vi "get_modelock_status.vi"(8 "error in (no error)":errorcluster, 11 "VISA resource name":refnum<visa-resource-name>) -> (0 "error out":errorcluster, 1 "color":u32, 2 "modelock (0,1,2=off,ML,CW)":i32, 3 "VISA resource name out":refnum<visa-resource-name>)   [LabVIEW 2013]
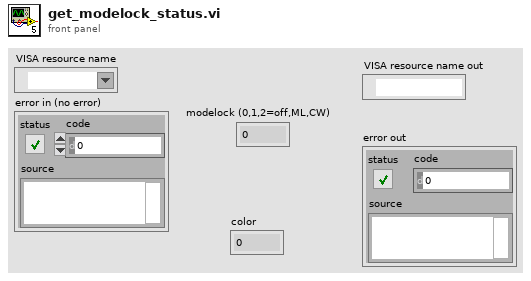
[diagram p1: front panel]
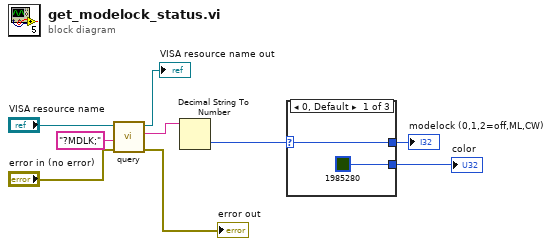
[diagram p0: block diagram]
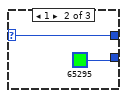
[diagram p2: hidden frame]
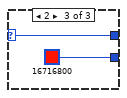
[diagram p3: hidden frame]
diagram:
  n1 = call "query.vi"("error in (no error)"="error in (no error)", "write buffer"="?MDLK;", "VISA resource name"="VISA resource name") -> ("error out"=→"error out":errorcluster, "substring"=w4:string, "VISA resource name out"=→"VISA resource name out":refnum<visa-resource-name>)  [unwired: 6 in]
  n2 = Decimal String To Number(string=w4) -> (number=w3:i32)  [unwired: 2 in, 1 out]
  n3 = case shown="0, Default" w3 {
    selector: w3 -> [w11 w13 w15]
    tunnel: [w11 w13 w15] -> w2
    tunnel: [u32 1985280 u32 65295 u32 16716800] -> w1
    frame 0, Default {
    }
    frame 1 {
    }
    frame 2 {
    }
  }
  "modelock (0,1,2=off,ML,CW)" <- w2
  "color" <- w1
